vi "getName.vi"(8 "error in (no error)":errorcluster, 11 "tBSONElement in":refnum<class "tBSONElement.lvclass">) -> (0 "error out":errorcluster, 2 "Name":string, 3 "tBSONElement out":refnum<class "tBSONElement.lvclass">)   [LabVIEW 2013, in "BSON.lvlib" / "tBSONElement.lvclass"]
uses:
  tBSONElement.lvclass
  tBSONElement.lvclass/tBSONElement.ctl
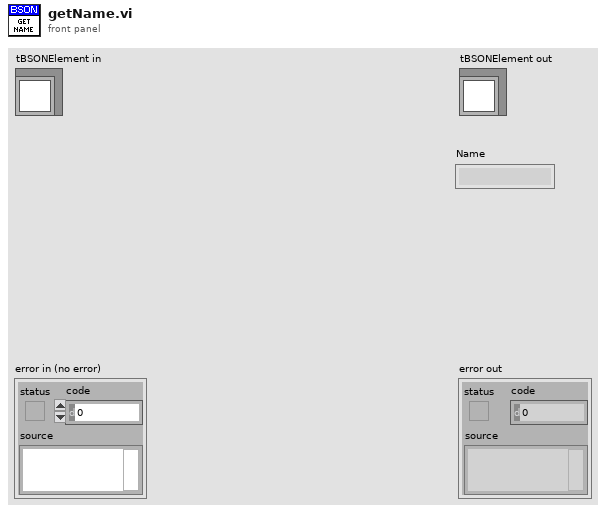
[diagram p1: front panel]
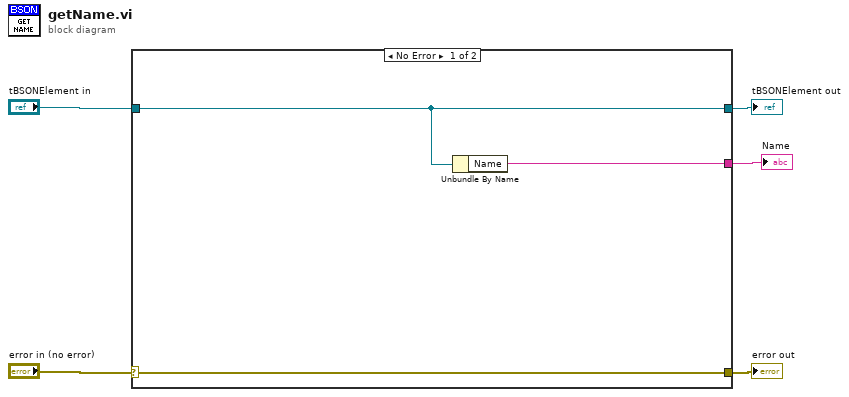
[diagram p0: block diagram]
diagram:
  n1 = case shown="No Error" "error in (no error)" {
    selector: "error in (no error)" -> [w8 w10]
    tunnel: [w8 w10] -> w4
    tunnel: [w7 w9] -> w2
    tunnel: "tBSONElement in" -> [w7 w9]
    tunnel: [w6 _] -> w1
    frame No Error {
      n2 = Unbundle By Name(w7) -> ("Name"=w6:string)
    }
    frame Error {
    }
  }
  "error out" <- w4
  "tBSONElement out" <- w2
  "Name" <- w1
